vi "getWfFromFile.vi"(8 "error in (no error)":errorcluster, 10 "Wfs Err Data":path=path "/home/ttsai/Documents/stash/ts_tcs_ofc/testData/lsst_wfs_error_iter0.z4c", 11 "ZTAAC in":refnum<class "ZTAAC.lvclass">) -> (0 "error out":errorcluster, 2 "Wavefront Error":dbl[][](array[numeric]), 3 "ZTAAC out":refnum<class "ZTAAC.lvclass">)   [LabVIEW 2016, in "OfcFunc.lvlib" / "ZTAAC.lvclass"]
doc: "Get the wavefront error from the file."
uses:
  ZTAAC.lvclass
  ZTAAC.lvclass/ZTAAC.ctl
  OptStateEsti/OptStateEsti.lvclass
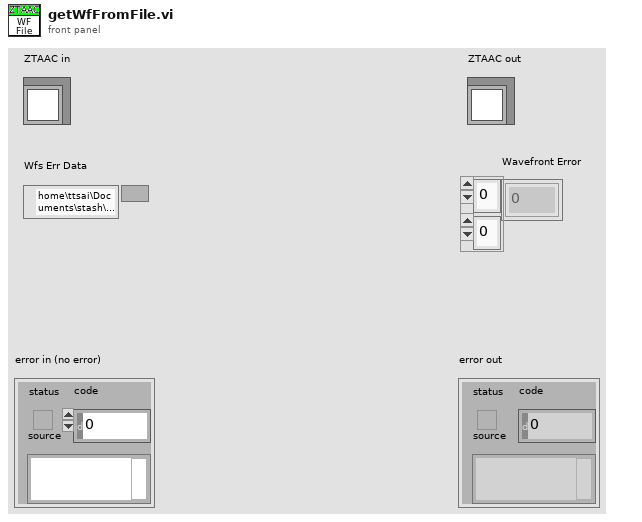
[diagram p1: front panel]
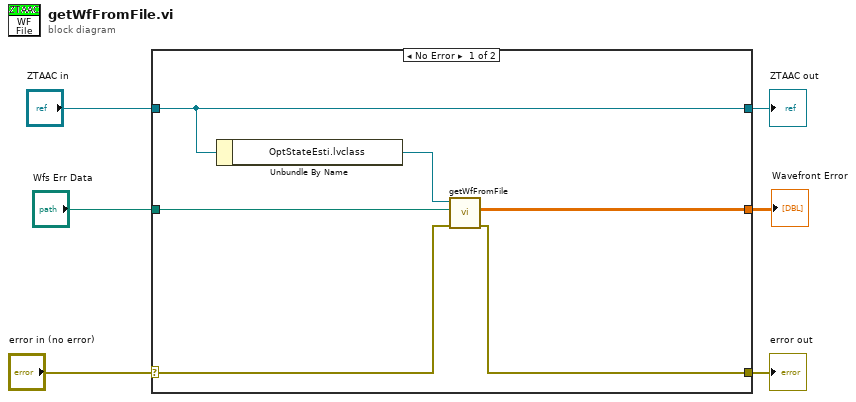
[diagram p0: block diagram]
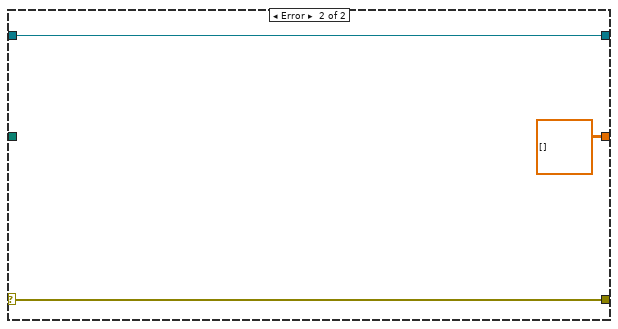
[diagram p2: hidden frame]
diagram:
  n1 = case shown="No Error" "error in (no error)" {
    selector: "error in (no error)" -> [w8 w15]
    tunnel: [w7 w15] -> w5
    tunnel: [w12 w14] -> w3
    tunnel: "ZTAAC in" -> [w12 w14]
    tunnel: "Wfs Err Data" -> [w10 _]
    tunnel: [w9 dbl[][] [] ("Matrix")] -> w1
    frame No Error {
      n2 = Unbundle By Name(w12) -> ("OptStateEsti.lvclass"=w11:refnum<class "OptStateEsti.lvclass">)
      n3 = call "getWfFromFile.vi"("error in (no error)"=w8, "Wfs Err Data"=w10, "OptStateEsti in"=w11) -> ("error out"=w7:errorcluster, "Wavefront Error"=w9:dbl[][])  [unwired: 5 in, 2 out]
    }
    frame Error {
    }
  }
  "error out" <- w5
  "ZTAAC out" <- w3
  "Wavefront Error" <- w1
